vi "EF_getAWTFeatures.vi"(9 "High cutoff frequency":dbl, 10 "Low cutoff frequency":dbl, 11 "Array Of Waveforms in":waveform(dbl)[](array[waveform])) -> (2 "size(s)":i32[](array[numeric]), 3 "MatrixOfMeanPowers":dbl[][](array[numeric]))   [LabVIEW 2016, in "Feature Extraction.lvlib"]
uses:
  <vilib>/Analysis/baseanly.llb/Mean (DBL).vi
  <vilib>/addons/Wavelet Analysis/continuous wavelet transform.llb/WA Analytic Wavelet Transform (Waveform).vi
  Feature Extraction.lvlib
  <vilib>/addons/_Advanced Signal Processing/NI_AdvSigProcTFA.lvlib
  <vilib>/addons/_Advanced Signal Processing/NI_AdvSigProcWA.lvlib
  <vilib>/Analysis/NI_AALBase.lvlib
panel:
  # "This VI is a part of BCI Design library, http://www.ru-bci.org \nCopyright © 2020, Sotnikov Peter, All rights reserved. License: GNU GPLv3"
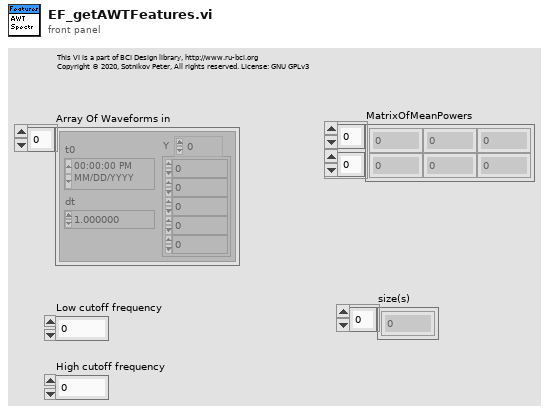
[diagram p1: front panel]
types:
  T1 = cluster{"frequency offset":dbl, "frequency multiplier":dbl}
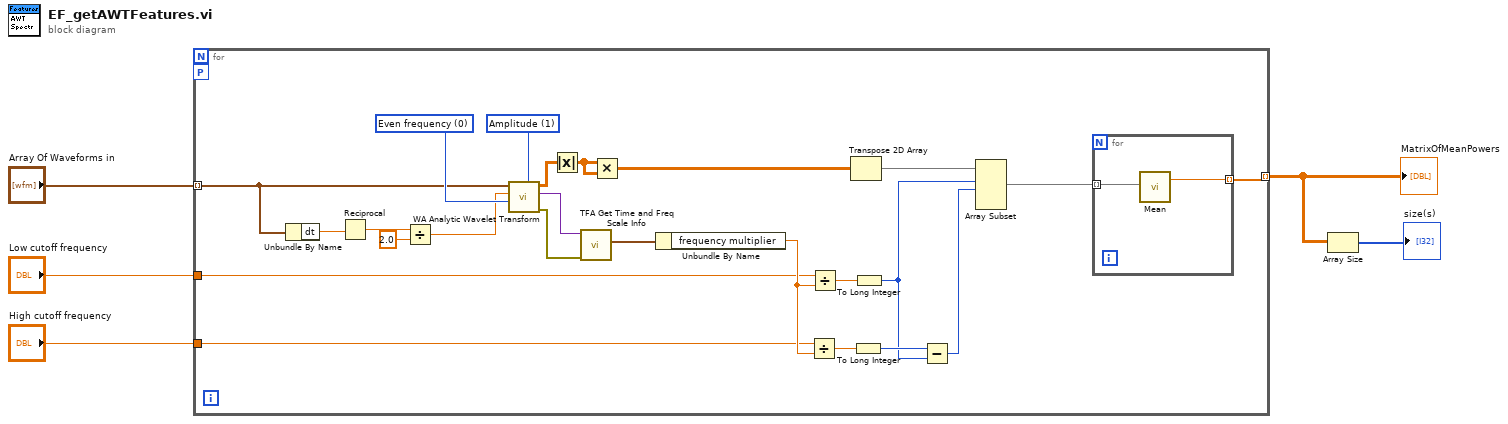
[diagram p0: block diagram]
diagram:
  n1 = for {
    tunnel: "Array Of Waveforms in" -> [w14] mode=indexing
    tunnel: [w8] -> w4 mode=indexing
    workers-P: _ -> [_]
    tunnel: "Low cutoff frequency" -> [w7]
    tunnel: "High cutoff frequency" -> [w6]
    w25 = u16 0 items=["Even frequency", "Even scale"] ("scale sampling method")
    w26 = u16 1 items=["Energy", "Amplitude"] ("normalization")
    n2 = Unbundle By Name(w14) -> ("dt"=w13:dbl)
    n3 = Reciprocal(x=w13) -> (1/x=w12:dbl)
    n4 = Divide(x=w12, y=2.0) -> (x/y=w10:dbl)
    n5 = call-poly <vilib>:"WA Analytic Wavelet Transform.vi"("normalization"=w26, "scale sampling method"=w25, "scales"=w10, "signal"=w14) -> ("error out"=w29:errorcluster, "scale info"=w27:variant, "AWT coef"=w24:cdb[][])  [unwired: 5 in]
    n6 = Absolute Value(x=w24) -> (abs(x)=w23:dbl[][])
    n7 = call <vilib>:"TFA Get Time and Freq Scale Info.vi"("error in (no error)"=w29, "scale info"=w27) -> ("frequency info"=w28:T1)  [unwired: 7 in, 2 out]
    n8 = Multiply(x=w23, y=w23) -> (x*y=w15:dbl[][])
    n9 = Unbundle By Name(w28) -> ("frequency multiplier"=w19:dbl)
    n10 = Divide(x=w6, y=w19) -> (x/y=w22:dbl)
    n11 = Divide(x=w7, y=w19) -> (x/y=w20:dbl)
    n12 = Transpose 2D Array(2D array=w15) -> (transposed array=w21:dbl[][])
    n13 = To Long Integer(number=w22) -> (32bit integer=w18:i32)
    n14 = To Long Integer(number=w20) -> (32bit integer=w17:i32)
    n15 = Subtract(x=w18, y=w17) -> (x-y=w16:i32)
    n16 = Array Subset(array=w21, index (row)=w17, length (row)=w16) -> (w9:dbl[][])  [unwired: 2 in]
    n17 = for {
      tunnel: w9 -> [w31] mode=indexing
      tunnel: [w30] -> w8 mode=indexing
      n18 = call-poly <vilib>:"Mean.vi"("X"=w31) -> ("mean"=w30:dbl)  [unwired: 1 out]
    }
  }
  "MatrixOfMeanPowers" <- w4
  n19 = Array Size(array=w4) -> (size(s)=→"size(s)":i32[])
